vi "calibrateWaveplatePhotons.vi"() -> ()   [LabVIEW 2013]
uses:
  <vilib>/Utility/file.llb/Write To Spreadsheet File (DBL).vi
panel:
  in  "Report":enum16{"Time to reach count", "Trigger rate"}(ring)
  in  "Start position":dbl
  out "Data":dbl[][](array[numeric])
  in  "Write to file?":bool
  out "error out":errorcluster
  in  "Photon number":dbl
  in  "Repetitions":dbl=1.0
  in  "file path (dialog if empty)":path
  out "XY Graph":cluster{"Y":dbl[], "Y":dbl[]}[](graph)
  in  "Stop position":dbl=180.0
  in  "Rotation increment":dbl=10.0 format="%.2f"
  out "Current position (units)":dbl format="%.2f"
  in  "Axis in":i32=3
  in  "Timeout (ms)":u32=500
  in  "SerialPort":u8=3
  in  "stop":bool
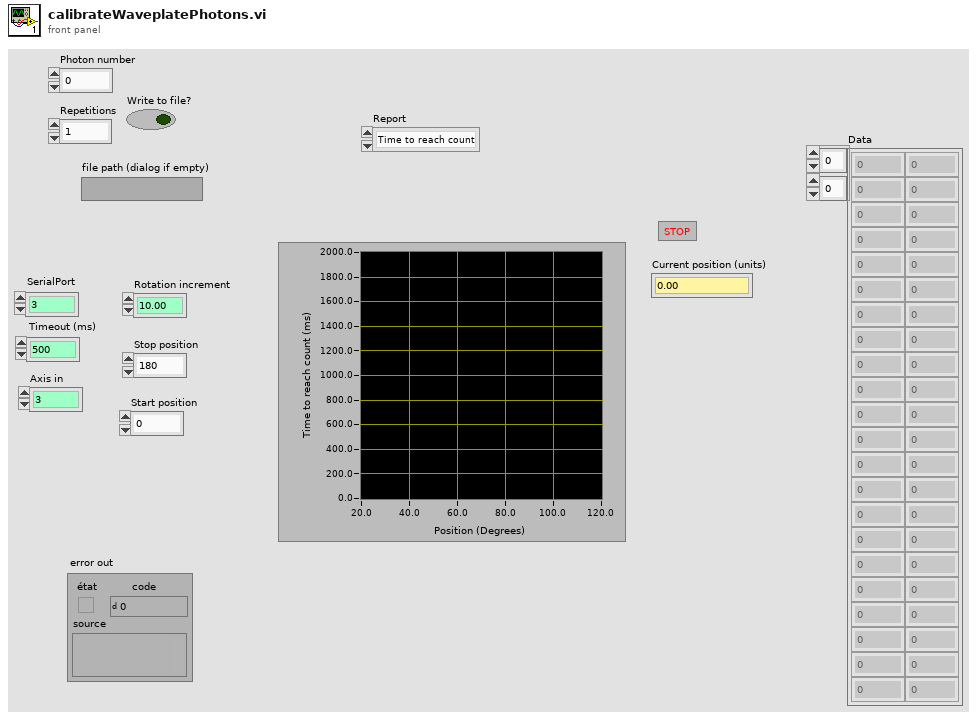
[diagram p1: front panel]
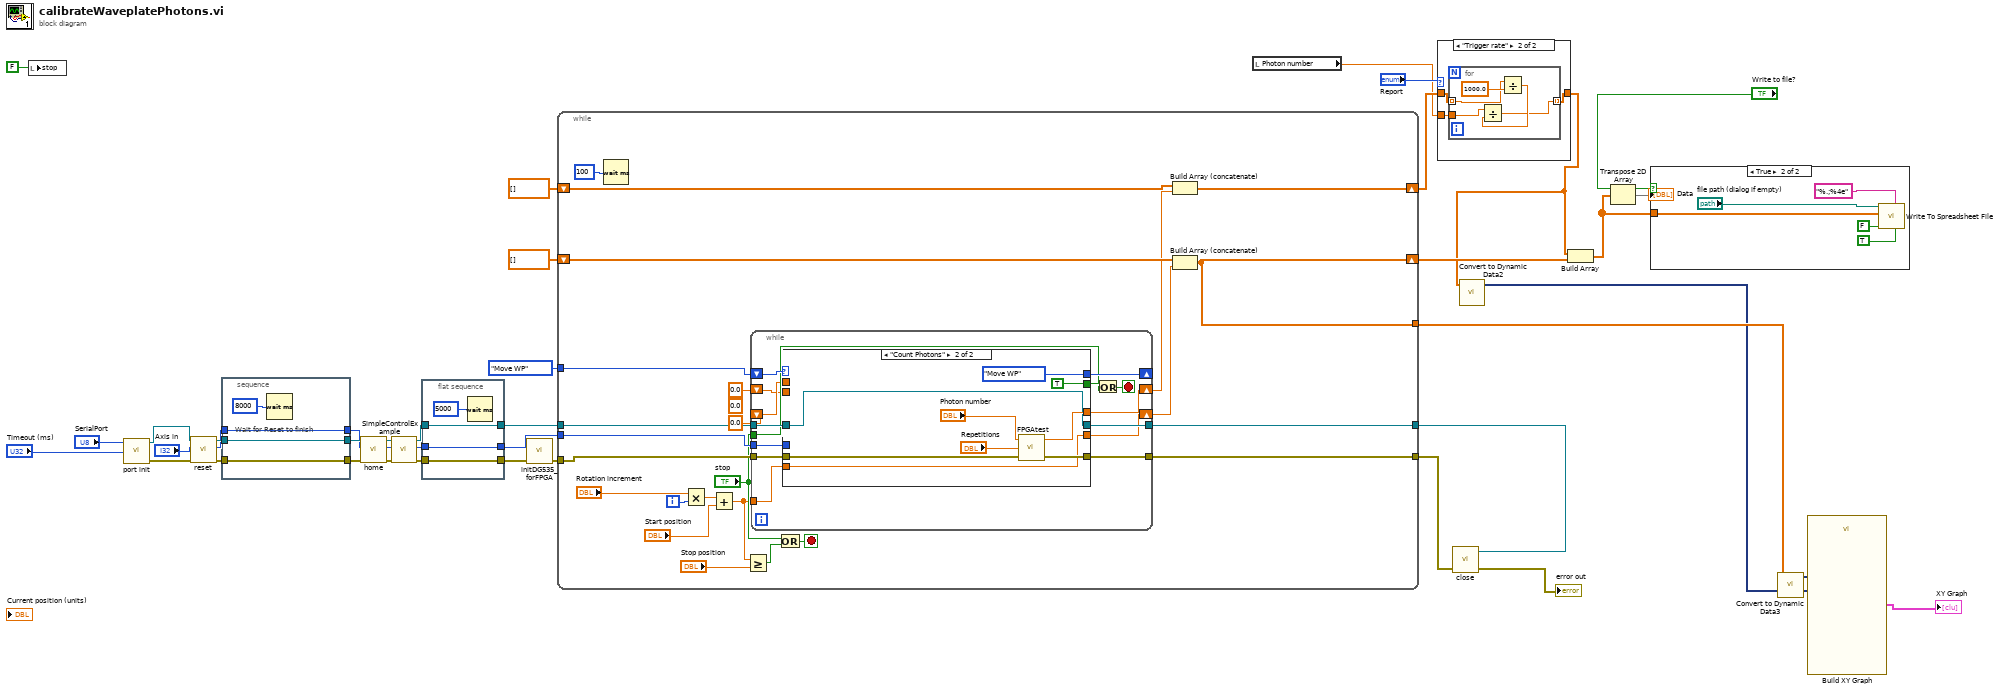
[diagram p0: block diagram]
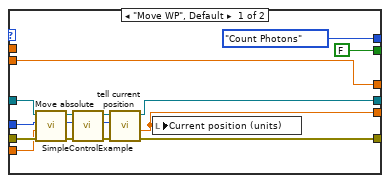
[diagram p4: hidden frame]
diagram:
  n1 = local write "stop"(FALSE ("stop")) -> ()
  n2 = call "port init.vi"("Timeout (ms)"="Timeout (ms)", "SerialPort"="SerialPort") -> ("error out"=w34:errorcluster, "Visa Handle"=w33:refnum<visa-resource-name>)  [unwired: 2 in]
  n3 = call "reset.vi"("error in"=w34, "Axis in"="Axis in", "VISA Handle in"=w33) -> ("error out"=w31:errorcluster, "Axis out"=w26:i32, "VISA Handle out"=w28:refnum<visa-resource-name>)  [unwired: 3 in, 1 out]
  n4 = stacked-sequence {
    tunnel: w31 -> [w43]
    tunnel: [w43] -> w30
    tunnel: [w42] -> w27
    tunnel: w28 -> [w42]
    tunnel: w26 -> [w41]
    tunnel: [w41] -> w25
    frame #0 {
      # "Wait for Reset to finish"
      n5 = Wait (ms)(milliseconds to wait=u32 8000) -> ()  [unwired: 1 out]
    }
  }
  n6 = call "home.vi"("error in"=w30, "Axis in"=w25, "VISA Handle in"=w27) -> ("error out"=w36:errorcluster, "Axis out"=w35:i32, "VISA Handle out"=w37:refnum<visa-resource-name>)  [unwired: 3 in, 1 out]
  n7 = call "SimpleControlExample.vi"("error in"=w36, "Axis in"=w35, "VISA Handle in"=w37) -> ("error out"=w20:errorcluster, "Axis out"=w24:i32, "VISA Handle out"=w22:refnum<visa-resource-name>)  [unwired: 2 in, 2 out]
  n8 = flat-sequence {
    tunnel: w24 -> [w48]
    tunnel: [w48] -> w23
    tunnel: w22 -> [w47]
    tunnel: [w47] -> w21
    tunnel: w20 -> [w46]
    tunnel: [w46] -> w15
    frame #0 {
      n9 = Wait (ms)(milliseconds to wait=u32 5000) -> ()  [unwired: 1 out]
    }
  }
  n10 = call "initDG535_forFPGA.vi"("error in"=w15) -> ("error out"=w14:errorcluster)  [unwired: 4 in]
  n11 = while {
    tunnel: enum16{"Move WP", "Count Photons", "Stop"}."Move WP" -> [w72]
    tunnel: w21 -> [w71]
    tunnel: w23 -> [w70]
    tunnel: w14 -> [w69]
    tunnel: [w63] -> w29
    tunnel: [w62] -> w18
    shift-right: [w50] -> w3
    shift-left: dbl[] [] -> [w59]
    shift-right: [w49] -> w13
    shift-left: dbl[] [] -> [w57]
    tunnel: [w49] -> w8
    i -> [w61]
    stop <- w64 stop-if-true
    (unwired) 0.0 ("Photon number")
    n12 = Wait (ms)(milliseconds to wait=u32 100) -> ()  [unwired: 1 out]
    n13 = Multiply(x="Rotation increment", y=w61) -> (x*y=w55:dbl)
    n14 = Add(x=w55, y="Start position") -> (x+y=w53:dbl)
    n15 = Greater Or Equal?(x=w53, y="Stop position") -> (x >= y?=w66:bool)
    n16 = while {
      shift-right: [w86] -> _
      shift-left: w72 -> [w87]
      tunnel: w71 -> [w85]
      tunnel: w70 -> [w84]
      tunnel: w69 -> [w83]
      tunnel: [w82] -> w62
      tunnel: [w81] -> w63
      tunnel: w53 -> [w78]
      tunnel: "stop" -> [w77]
      shift-right: [w76] -> w58
      shift-left: 0.0 ("Current position (units)") -> [w75]
      shift-right: [w74] -> w56
      shift-left: 0.0 ("Value") -> [w73]
      stop <- w79 stop-if-true
      n17 = case shown="\"Count Photons\"" w87 {
        tunnel: [enum16{"Move WP", "Count Photons", "Stop"}."Count Photons" enum16{"Move WP", "Count Photons", "Stop"}."Move WP"] -> w86
        tunnel: w85 -> [w97 w106]
        tunnel: w84 -> [w96 _]
        tunnel: w83 -> [w95 w111]
        tunnel: [w94 w110] -> w82
        tunnel: [w93 w106] -> w81
        tunnel: [FALSE ("x") TRUE ("x")] -> w80
        tunnel: w78 -> [w91 w105]
        tunnel: [w90 w105] -> w76
        tunnel: w75 -> [_ _]
        tunnel: [w88 w109] -> w74
        tunnel: w73 -> [w88 _]
        frame "Move WP", Default {
          n18 = call "Move absolute.vi"("error in"=w95, "New target position (units)"=w91, "Axis in"=w96, "VISA Handle in"=w97) -> ("error out"=w98:errorcluster, "Axis out"=w99:i32, "VISA Handle out"=w100:refnum<visa-resource-name>)  [unwired: 2 in, 1 out]
          n19 = call "SimpleControlExample.vi"("error in"=w98, "Axis in"=w99, "VISA Handle in"=w100) -> ("error out"=w101:errorcluster, "Axis out"=w102:i32, "VISA Handle out"=w103:refnum<visa-resource-name>)  [unwired: 2 in, 2 out]
          n20 = call "tell current position.vi"("error in"=w101, "Axis in"=w102, "VISA Handle in"=w103) -> ("error out"=w94:errorcluster, "Current position (units)"=w90:dbl, "VISA Handle out"=w93:refnum<visa-resource-name>)  [unwired: 2 in, 2 out]
          n21 = local write "Current position (units)"(w90) -> ()
        }
        frame "Count Photons" {
          n22 = call "FPGAtest.vi"("Error in"=w111, "Repetitions"="Repetitions", "Photon number"="Photon number") -> ("Error out"=w110:errorcluster, "Value"=w109:dbl)  [unwired: 1 in]
        }
      }
      n23 = Or(x=w80, y=w77) -> (x .or. y?=w79:bool)
    }
    n24 = Or(x="stop", y=w66) -> (x .or. y?=w64:bool)
    n25 = Build Array (concatenate)(w59, w56) -> (w50:dbl[])
    n26 = Build Array (concatenate)(w57, w58) -> (w49:dbl[])
  }
  n27 = local read "Photon number"() -> (w1:dbl)
  n28 = case shown="\"Trigger rate\"" "Report" {
    tunnel: w3 -> [w113 w116]
    tunnel: [w113 w115] -> w2
    tunnel: w1 -> [_ w114]
    frame "Time to reach count", Default {
    }
    frame "Trigger rate" {
      n29 = for {
        tunnel: w116 -> [w120] mode=indexing
        tunnel: [w118] -> w115 mode=indexing
        tunnel: w114 -> [w117]
        n30 = Divide(x=w120, y=1000.0) -> (x/y=w119:dbl)
        n31 = Divide(x=w117, y=w119) -> (x/y=w118:dbl)
      }
    }
  }
  n32 = call "close.vi"("error in"=w18, "VISA Handle in"=w29) -> ("error out"=→"error out":errorcluster)  [unwired: 3 in]
  n33 = call "Convert to Dynamic Data2"("Array"=w2) -> ("Dynamic Data Type"=w6:dynamicdata)  [unwired: 3 in]
  n34 = Build Array(w2, w13) -> (w11:dbl[][])
  n35 = Transpose 2D Array(2D array=w11) -> (transposed array=→"Data":dbl[][])
  n36 = case shown="True" "Write to file?" {
    tunnel: w11 -> [_ w122]
    frame False {
    }
    frame True {
      n37 = call-poly <vilib>:"Write To Spreadsheet File.vi"("transpose? (no:F)"=TRUE, "format (%.3f)"="%.;%4e", "append to file? (new file:F)"=FALSE, "2D data"=w122, "file path (dialog if empty)"="file path (dialog if empty)") -> ()  [unwired: 3 in, 1 out]
    }
  }
  n38 = call "Convert to Dynamic Data3"("Array"=w8) -> ("Dynamic Data Type"=w4:dynamicdata)  [unwired: 3 in]
  n39 = call "Build XY Graph"("Y Input"=w6, "X Input"=w4) -> ("XY Graph"=→"XY Graph":cluster{"Y":dbl[], "Y":dbl[]}[])  [unwired: 3 in, 6 out]
